vi "Update FPGA Parameters.vi"(8 "error in":errorcluster, 11 "cPAS in":refnum<class "cPAS.lvclass">) -> (0 "error out":errorcluster, 2 "Update FPGA?":bool, 3 "cPAS out":refnum<class "cPAS.lvclass">)   [LabVIEW 2015]
uses:
  Instruments/AOP/cPAS.lvclass
  PAS/Main/Controls/Laser Modulation.ctl
  Instruments/AOP/cPAS.lvclass/cPAS.ctl
  PAS/Main/PAS.lvclass
  PAS/Cell/PAS Cell.lvclass
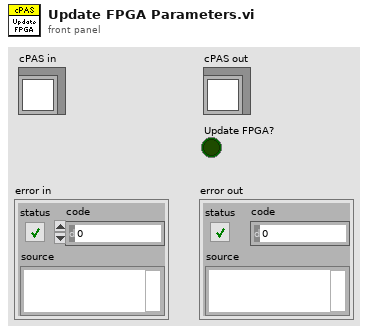
[diagram p1: front panel]
types:
  T1 = typedef "Laser Modulation.ctl" = enum8{"Sine", "Square"}
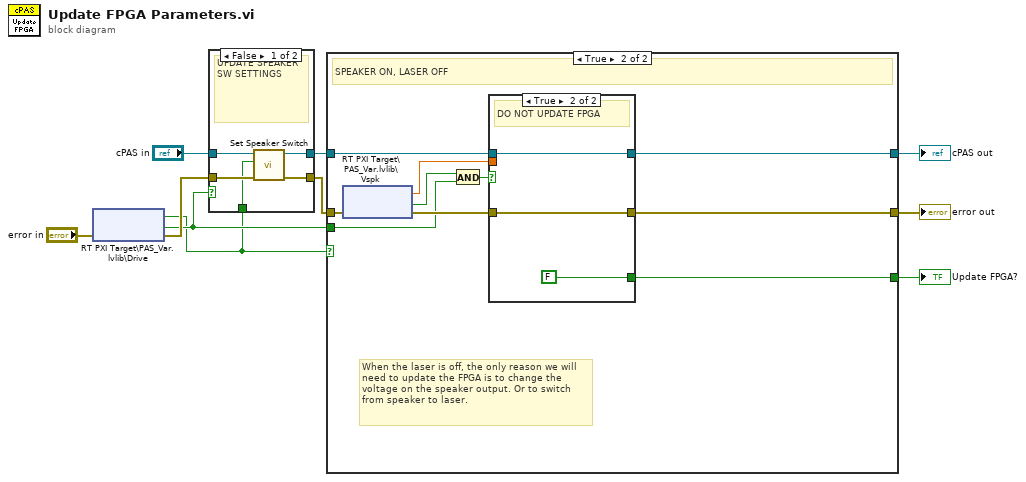
[diagram p0: block diagram]
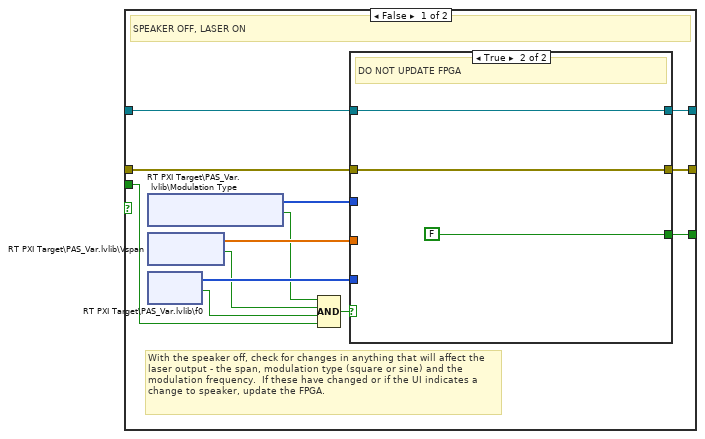
[diagram p2: hidden frame]
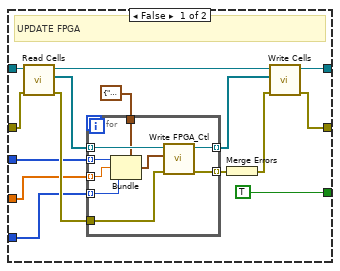
[diagram p3: hidden frame]
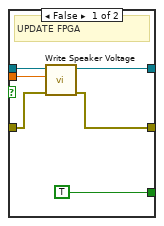
[diagram p4: hidden frame]
diagram:
  n1 = shared-variable "RT PXI Target\\PAS_Var.lvlib\\Drive"(error in="error in") -> (w1:bool, error out=w6:errorcluster, w2:bool)  [unwired: 1 in]
  n2 = case shown="False" w2 {
    tunnel: "cPAS in" -> [w15 w17]
    tunnel: w6 -> [w14 w16]
    tunnel: [w13 w17] -> w7
    tunnel: [w12 w16] -> w5
    tunnel: w1 -> [w11 _]
    frame False {
      # "UPDATE SPEAKER SW SETTINGS"
      n3 = call "Set Speaker Switch.vi"("error in"=w14, "State"=w11, "PAS in"=w15) -> ("error out"=w12:errorcluster, "PAS out"=w13:refnum<class "cPAS.lvclass">)  [unwired: 7 in]
    }
    frame True {
    }
  }
  n4 = case shown="True" w1 {
    tunnel: w7 -> [w30 w65]
    tunnel: w5 -> [w19 w64]
    tunnel: w2 -> [w24 w59]
    tunnel: [w22 w62] -> w4
    tunnel: [w21 w63] -> w3
    tunnel: [w18 w61] -> w9
    frame False {
      # "With the speaker off, check for changes in anything that will affect the laser output - the span, modulation type (square or sine) and the modulation frequency.  If these have changed or if the UI indicates a change to speaker, update the FPGA."
      # "SPEAKER OFF, LASER ON"
      n5 = shared-variable "RT PXI Target\\PAS_Var.lvlib\\Modulation Type"() -> (w29:u8[], w26:bool)  [unwired: 2 in, 1 out]
      n6 = shared-variable "RT PXI Target\\PAS_Var.lvlib\\Vspan"() -> (w28:sgl[], w20:bool)  [unwired: 2 in, 1 out]
      n7 = shared-variable "RT PXI Target\\PAS_Var.lvlib\\f0"() -> (w27:u16[], w25:bool)  [unwired: 2 in, 1 out]
      n8 = Compound Arithmetic op=AND(w26, w20, w25, w24) -> (w23:bool)
      n9 = case shown="True" w23 {
        tunnel: w30 -> [w41 w57]
        tunnel: w29 -> [w40 _]
        tunnel: w28 -> [w31 _]
        tunnel: w27 -> [w39 _]
        tunnel: [w36 w57] -> w22
        tunnel: [w33 w56] -> w21
        tunnel: w19 -> [w35 w56]
        tunnel: [TRUE FALSE] -> w18
        frame False {
          # "UPDATE FPGA"
          n10 = call "Read Cells.vi"("error in (no error)"=w35, "PAS in"=w41) -> ("error out"=w44:errorcluster, "Cells"=w45:refnum<class "PAS Cell.lvclass">[], "PAS out"=w38:refnum<class "cPAS.lvclass">)  [unwired: 7 in]
          n11 = for {
            tunnel: [w54] -> w37 mode=indexing
            tunnel: w45 -> [w53] mode=indexing
            tunnel: w39 -> [w46] mode=indexing
            tunnel: w31 -> [w51] mode=indexing
            tunnel: w40 -> [w52] mode=indexing
            tunnel: w44 -> [w50]
            tunnel: [w48] -> w43 mode=indexing
            tunnel: cluster{"Mod":T1, "Span":sgl, "f0":sgl} {"Mod"=enum."Sine", "Span"=0.0, "f0"=0.0} ("FPGA_Ctl") -> [w47]
            n12 = Bundle(cluster=w47, "Mod"=w52, "Span"=w51, "f0"=w46) -> (w49:cluster{"Mod":T1, "Span":sgl, "f0":sgl})
            n13 = call "Write FPGA_Ctl.vi"("error in (no error)"=w50, "FPGA_Ctl"=w49, "PAS Cell in"=w53) -> ("error out"=w48:errorcluster, "PAS Cell out"=w54:refnum<class "PAS Cell.lvclass">)  [unwired: 7 in]
          }
          n14 = Merge Errors(w43) -> (w34:errorcluster)
          n15 = call "Write Cells.vi"("error in"=w34, "Cells"=w37, "PAS in"=w38) -> ("error out"=w33:errorcluster, "PAS out"=w36:refnum<class "cPAS.lvclass">)  [unwired: 7 in]
        }
        frame True {
          # "DO NOT UPDATE FPGA"
        }
      }
    }
    frame True {
      # "When the laser is off, the only reason we will need to update the FPGA is to change the voltage on the speaker output. Or to switch from speaker to laser."
      # "SPEAKER ON, LASER OFF"
      n16 = shared-variable "RT PXI Target\\PAS_Var.lvlib\\Vspk"(error in=w64) -> (w67:sgl, error out=w66:errorcluster, w60:bool)  [unwired: 1 in]
      n17 = And(x=w60, y=w59) -> (x .and. y?=w58:bool)
      n18 = case shown="True" w58 {
        tunnel: w65 -> [w73 w76]
        tunnel: [w72 w76] -> w62
        tunnel: w66 -> [w71 w75]
        tunnel: [w70 w75] -> w63
        tunnel: w67 -> [w69 _]
        tunnel: [TRUE FALSE] -> w61
        frame False {
          # "UPDATE FPGA"
          n19 = call "Write Speaker Voltage.vi"("error in (no error)"=w71, "Speaker Voltage"=w69, "cPAS in"=w73) -> ("error out"=w70:errorcluster, "cPAS out"=w72:refnum<class "cPAS.lvclass">)  [unwired: 7 in]
        }
        frame True {
          # "DO NOT UPDATE FPGA"
        }
      }
    }
  }
  "error out" <- w3
  "cPAS out" <- w4
  "Update FPGA?" <- w9
